vi "unmarshalling.vi"(7 "Type":variant, 8 "error in (no error)":errorcluster, 10 "JSON String":string, 11 "Serializer":refnum<class "Serializer.JSON.lvclass">) -> (0 "error out":errorcluster, 2 "Variant":variant, 3 "Serializer out":refnum<class "Serializer.JSON.lvclass">)   [LabVIEW 2019, in "OpenSerializer.JKI-JSON.lvlib" / "Serializer.JSON.lvclass"]
uses:
  Serializer.JSON.lvclass
  <vilib>/addons/_JKI.lib/Serialization/JSON/JKI JSON Serialization.lvlib
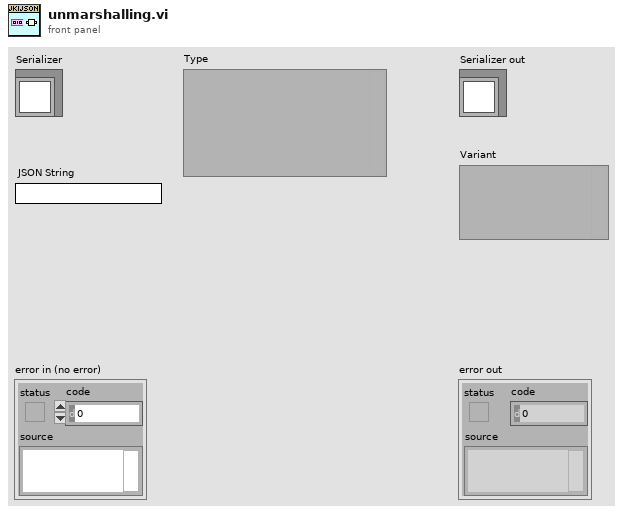
[diagram p1: front panel]
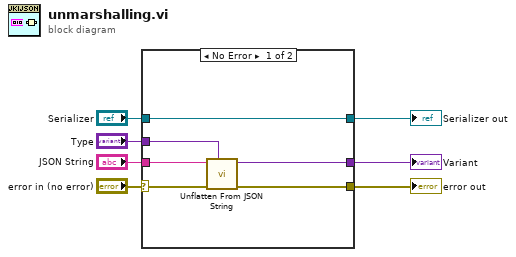
[diagram p0: block diagram]
diagram:
  n1 = case shown="No Error" "error in (no error)" {
    selector: "error in (no error)" -> [w11 w15]
    tunnel: "Serializer" -> [w9 w16]
    tunnel: "JSON String" -> [w12 _]
    tunnel: [w9 w16] -> w5
    tunnel: [w8 w15] -> w4
    tunnel: [w10 w14] -> w3
    tunnel: "Type" -> [w13 w14]
    frame No Error {
      n2 = call <vilib>:"Unflatten From JSON String.vi"("Type and Defaults"=w13, "error in (no error)"=w11, "JSON String"=w12) -> ("error out"=w8:errorcluster, "Variant"=w10:variant)  [unwired: 7 in]
    }
    frame Error {
    }
  }
  "error out" <- w4
  "Serializer out" <- w5
  "Variant" <- w3
